vi "项名.vi"(8 "error in (no error)":errorcluster caption="错误输入（无错误）", 11 "Delete 输入":refnum<class "Delete.lvclass">) -> (0 "error out":errorcluster caption="错误输出", 3 "Delete 输出":refnum<class "Delete.lvclass">)   [LabVIEW 2016, in "Delete.lvclass"]
uses:
  Delete.lvclass
  Parent Class/Menu.lvclass
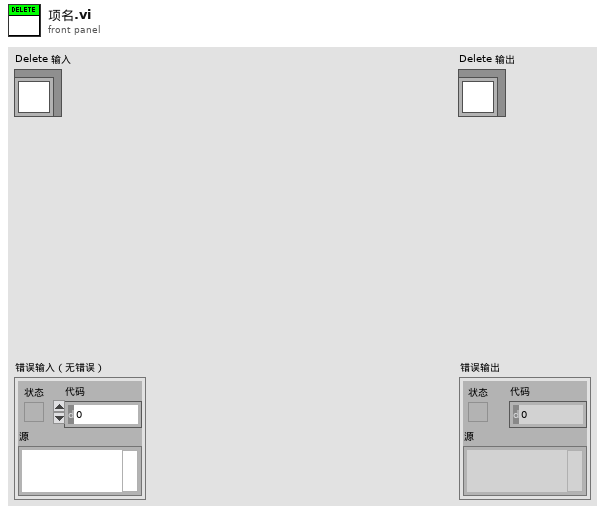
[diagram p1: front panel]
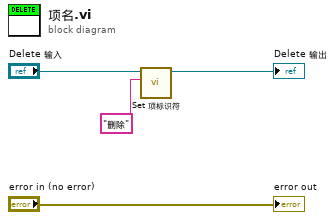
[diagram p0: block diagram]
diagram:
  n1 = call "Set 项标识符.vi"("项标识符"="删除", "LNK in"="Delete 输入") -> ("LNK out"=→"Delete 输出":refnum<class "Delete.lvclass">)  [unwired: 9 in]
  "error out" <- "error in (no error)"
